vi "test-trajectory-generate-01.vi"() -> ()   [LabVIEW 2019]
uses:
  <vilib>/Rock Robotics/WPI/ThirdParty/JAS_Junk/TrajLib/Trajectory_Library.lvlib
  <vilib>/Rock Robotics/WPI/ThirdParty/JAS_Junk/TrajLib/TypeDef/TRANSLATION2D.ctl
  <vilib>/Rock Robotics/WPI/ThirdParty/JAS_Junk/TrajLib/TypeDef/ROTATION2D.ctl
  <vilib>/Rock Robotics/WPI/ThirdParty/JAS_Junk/TrajLib/TypeDef/POSE2D.ctl
  <vilib>/Rock Robotics/WPI/ThirdParty/JAS_Junk/TrajLib/TypeDef/TRAJ_STATE.ctl
panel:
  out "Accel\nExceeded (F)":bool
  out "Speed\nExceeded  (F)":bool
  out "TotalTImeSecs":dbl
  out "States":T1[](array[typedef]) {"POSE"."ROTATION"."SIN" format="%13.4f"; "POSE"."ROTATION"."COS" format="%13.4f"; "POSE"."ROTATION"."VALUE" format="%13.4f"; "POSE"."TRANSLATION"."Y" format="%14.3f"; "POSE"."TRANSLATION"."X" format="%14.3f"}
  out "XY Graph":cluster{dbl[], dbl[]}(graph)
  out "Numb\nWaypoints":i32
  out "All Interior \nwayPoints\nFound (True)":bool
  out "end rot = 0":dbl
  out "end y = 0":dbl
  out "end x = 0":dbl
  out "start rot = 0":dbl
  out "start y = 0":dbl
  out "start x = 0":dbl
  out "max dtheta < 0.0872":dbl
  out "max dy < 0.00127":dbl
  out "max dx  < 0.127":dbl
  out "Overall Error":errorcluster
  out "Elements":i32
  out "Elapsed Time":dbl
  # "THIS TEST SHOULD FAIL"
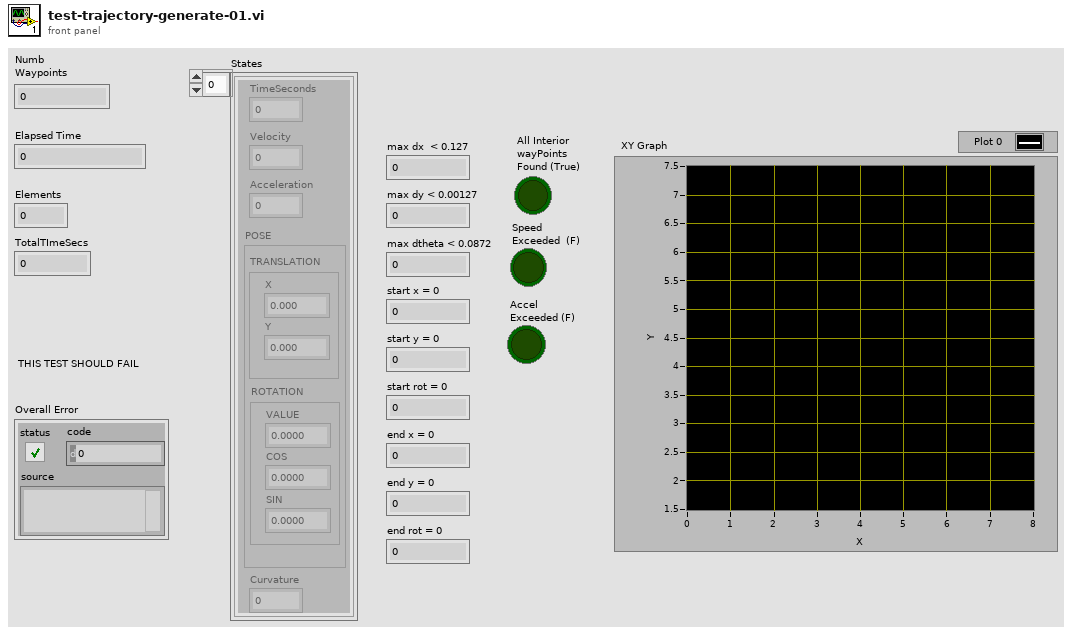
[diagram p1: front panel]
types:
  T1 = typedef "Trajectory_Library.lvlib/TRAJ_STATE.ctl" = cluster{"TimeSeconds":dbl, "Velocity":dbl, "Acceleration":dbl, "POSE":T2, "Curvature":dbl}
  T2 = typedef "Trajectory_Library.lvlib/POSE2D.ctl" = cluster{"TRANSLATION":T3, "ROTATION":T4}
  T3 = typedef "Trajectory_Library.lvlib/TRANSLATION2D.ctl" = cluster{"X":dbl, "Y":dbl}
  T4 = typedef "Trajectory_Library.lvlib/ROTATION2D.ctl" = cluster{"VALUE":dbl, "COS":dbl, "SIN":dbl}
  T5 = typedef "Trajectory_Library.lvlib/TRAJ_CONFIG.ctl" = cluster{"MaxVelocity":dbl, "Max Acceleration":dbl, "StartVelocity":dbl, "End Velocity":dbl, "Reversed":bool, "Constraints":variant[]}
  T6 = typedef "Trajectory_Library.lvlib/TRAJECTORY.ctl" = cluster{"TotalTImeSecs":dbl, "States":T1[]}
  T7 = typedef "Trajectory_Library.lvlib/TWIST2D.ctl" = cluster{"dX":dbl, "dY":dbl, "dTHETA":dbl}
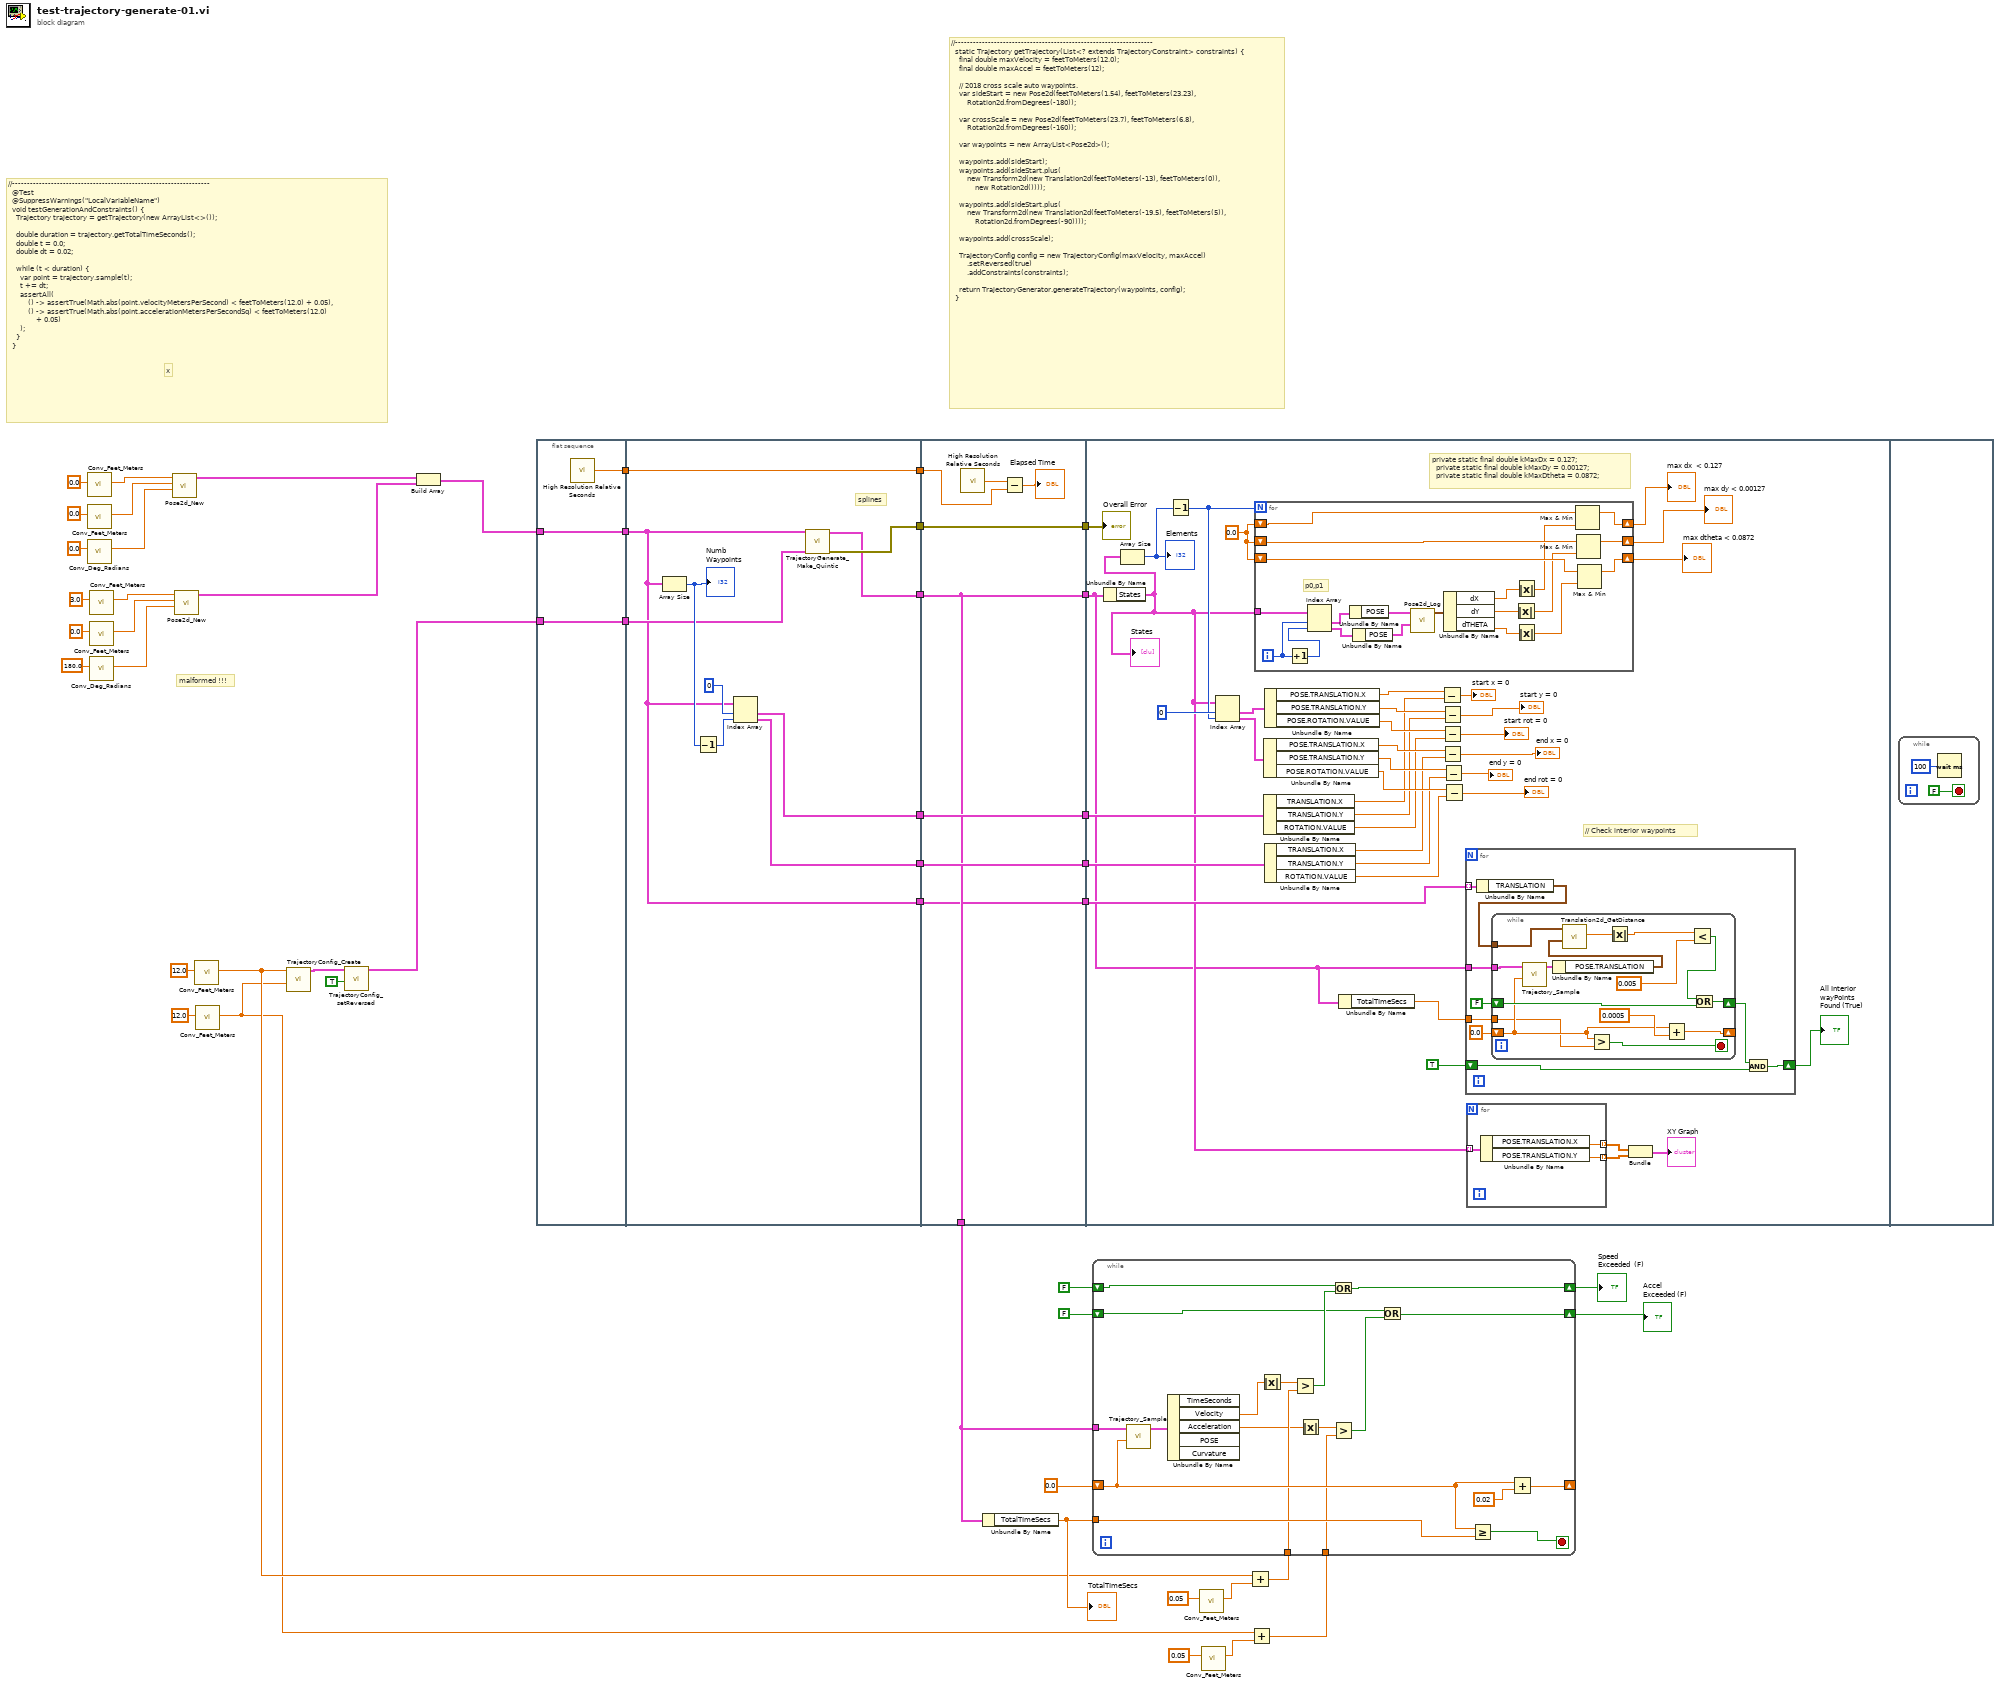
[diagram p0: block diagram]
diagram:
  # "malformed !!!"
  # "//------------------------------------------------------------------\n  @Test\n  @SuppressWarnings(\"LocalVariableName\")\n  void testGenerationAndConstraints() {\n    Trajectory trajectory = getTrajectory(new ArrayList<>());\n\n    double duration = trajectory.getTotalTimeSeconds();\n    double t = 0.0;\n    double dt = 0.02;\n\n    while (t < duration) {\n      var point = trajectory.sample(t);\n      t += dt;\n      assertAll(\n          () -> assertTrue(Math.abs(point.velocityMetersPerSecond) < feetToMeters(12.0) + 0.05),\n          () -> assertTrue(Math.abs(point.accelerationMetersPerSecondSq) < feetToMeters(12.0)\n              + 0.05)\n      );\n    }\n  }"
  # "//------------------------------------------------------------------\n  static Trajectory getTrajectory(List<? extends TrajectoryConstraint> constraints) {\n    final double maxVelocity = feetToMeters(12.0);\n    final double maxAccel = feetToMeters(12);\n\n    // 2018 cross scale auto waypoints.\n    var sideStart = new Pose2d(feetToMeters(1.54), feetToMeters(23.23),\n        Rotation2d.fromDegrees(-180));\n\n    var crossScale = new Pose2d(feetToMeters(23.7), feetToMeters(6.8),\n        Rotation2d.fromDegrees(-160));\n\n    var waypoints = new ArrayList<Pose2d>();\n\n    waypoints.add(sideStart);\n    waypoints.add(sideStart.plus(\n        new Transform2d(new Translation2d(feetToMeters(-13), feetToMeters(0)),\n            new Rotation2d())));\n\n    waypoints.add(sideStart.plus(\n        new Transform2d(new Translation2d(feetToMeters(-19.5), feetToMeters(5)),\n            Rotation2d.fromDegrees(-90))));\n\n    waypoints.add(crossScale);\n\n    TrajectoryConfig config = new TrajectoryConfig(maxVelocity, maxAccel)\n        .setReversed(true)\n        .addConstraints(constraints);\n\n    return TrajectoryGenerator.generateTrajectory(waypoints, config);\n  }"
  # "x"
  n1 = call <vilib>:"Conv_Feet_Meters.vi"("Feet"=0.0) -> ("Meters"=w39:dbl)  [unwired: 10 in]
  n2 = call <vilib>:"Conv_Feet_Meters.vi"("Feet"=0.0) -> ("Meters"=w38:dbl)  [unwired: 10 in]
  n3 = call <vilib>:"Conv_Deg_Radians.vi"("Degress"=0.0) -> ("Radians"=w37:dbl)  [unwired: 10 in]
  n4 = call <vilib>:"Conv_Feet_Meters.vi"("Feet"=3.0) -> ("Meters"=w33:dbl)  [unwired: 10 in]
  n5 = call <vilib>:"Conv_Feet_Meters.vi"("Feet"=0.0) -> ("Meters"=w32:dbl)  [unwired: 10 in]
  n6 = call <vilib>:"Conv_Deg_Radians.vi"("Degress"=180.0) -> ("Radians"=w31:dbl)  [unwired: 10 in]
  n7 = call <vilib>:"Pose2d_New.vi"("Heading"=w37, "Y"=w38, "X"=w39) -> ("out POSe"=w30:T2)  [unwired: 8 in]
  n8 = call <vilib>:"Pose2d_New.vi"("Heading"=w31, "Y"=w32, "X"=w33) -> ("out POSe"=w1:T2)  [unwired: 8 in]
  n9 = call <vilib>:"Conv_Feet_Meters.vi"("Feet"=12.0) -> ("Meters"=w14:dbl)  [unwired: 10 in]
  n10 = call <vilib>:"Conv_Feet_Meters.vi"("Feet"=12.0) -> ("Meters"=w4:dbl)  [unwired: 10 in]
  n11 = call <vilib>:"TrajectoryConfig_Create.vi"("MaxAcceleration"=w4, "MaxVelocity"=w14) -> ("TRAJECTORY_CONFIG"=w26:T5)  [unwired: 9 in]
  n12 = call <vilib>:"TrajectoryConfig_setReversed.vi"("Reversed"=TRUE, "inTRAJECTORY_CONFIG"=w26) -> ("outTRAJECTORY_CONFIG"=w22:T5)  [unwired: 9 in]
  n13 = Build Array(w30, w1) -> (w24:T2[])
  n14 = flat-sequence {
    tunnel: [w52] -> w49
    tunnel: [w51] -> w25
    tunnel: w24 -> [w51]
    tunnel: [w50] -> w23
    tunnel: w22 -> [w50]
    tunnel: [w62] -> w48
    tunnel: w49 -> [w62]
    tunnel: [w58] -> w46
    tunnel: [w57] -> w44
    tunnel: w25 -> [w53]
    tunnel: w23 -> [w54]
    tunnel: [w56] -> w21
    tunnel: [w55] -> w20
    tunnel: [w53] -> w2
    tunnel: w48 -> [w70]
    tunnel: [w65] -> w47
    tunnel: w46 -> [w67]
    tunnel: [w67] -> w45
    tunnel: w44 -> [w66]
    tunnel: [w66] -> w43
    tunnel: w21 -> [w65]
    tunnel: w20 -> [w64]
    tunnel: [w64] -> w19
    tunnel: [w64] -> w16
    tunnel: [w63] -> w3
    tunnel: w2 -> [w63]
    tunnel: w47 -> [w109]
    tunnel: w45 -> [w103]
    tunnel: w43 -> [w102]
    tunnel: w19 -> [w71]
    tunnel: w3 -> [w74]
    frame #0 {
      n15 = call <vilib>:"High Resolution Relative Seconds.vi"() -> ("relative seconds"=w52:dbl)
    }
    frame #1 {
      # "splines"
      n16 = Array Size(array=w53) -> (size(s)=w59:i32)
      "Numb\nWaypoints" <- w59
      n17 = Decrement(x=w59) -> (x-1=w60:i32)
      n18 = Index Array(array=w53, index #1=0 ("index"), index #2=w60) -> (element #1=w58:T2, element #2=w57:T2)
      n19 = call <vilib>:"TrajectoryGenerate_Make_Quintic.vi"("traj_config"=w54, "waypointPOSE"=w53) -> ("error out"=w56:errorcluster, "TRAJECTORY"=w55:T6)  [unwired: 8 in]
    }
    frame #2 {
      n20 = call <vilib>:"High Resolution Relative Seconds.vi"() -> ("relative seconds"=w68:dbl)
      n21 = Subtract(x=w68, y=w70) -> (x-y=→"Elapsed Time":dbl)
    }
    frame #3 {
      w107 = 0.0
      # "// Check interior waypoints"
      # "private static final double kMaxDx = 0.127;\n  private static final double kMaxDy = 0.00127;\n  private static final double kMaxDtheta = 0.0872;"
      n22 = Unbundle By Name(w71) -> ("States"=w72:T1[])
      "States" <- w72
      n23 = Array Size(array=w72) -> (size(s)=w108:i32)
      "Elements" <- w108
      n24 = Decrement(x=w108) -> (x-1=w100:i32)
      n25 = Index Array(array=w72, index #1=0 ("index"), index #2=w100) -> (element #1=w99:T1, element #2=w98:T1)
      n26 = for {
        N: w100 -> [_]
        tunnel: w72 -> [w154]
        shift-right: [w145] -> w106
        shift-left: w107 -> [w142]
        shift-right: [w143] -> w104
        shift-left: w107 -> [w140]
        shift-right: [w144] -> w105
        shift-left: w107 -> [w141]
        i -> [w156]
        # "p0,p1"
        n27 = Increment(x=w156) -> (x+1=w155:i32)
        n28 = Index Array(array=w154, index #1=w156, index #2=w155) -> (element #1=w153:T1, element #2=w152:T1)
        n29 = Unbundle By Name(w153) -> ("POSE"=w151:T2)
        n30 = Unbundle By Name(w152) -> ("POSE"=w150:T2)
        n31 = call <vilib>:"Pose2d_Log.vi"("end POSE"=w150, "in POSE"=w151) -> ("out TWIST"=w149:T7)  [unwired: 9 in]
        n32 = Unbundle By Name(w149) -> ("dX"=w146:dbl, "dY"=w147:dbl, "dTHETA"=w148:dbl)
        n33 = Absolute Value(x=w147) -> (abs(x)=w138:dbl)
        n34 = Absolute Value(x=w146) -> (abs(x)=w139:dbl)
        n35 = Absolute Value(x=w148) -> (abs(x)=w137:dbl)
        n36 = Max & Min(x=w142, y=w139) -> (max(x,y)=w145:dbl)  [unwired: 1 out]
        n37 = Max & Min(x=w141, y=w138) -> (max(x,y)=w144:dbl)  [unwired: 1 out]
        n38 = Max & Min(x=w140, y=w137) -> (max(x,y)=w143:dbl)  [unwired: 1 out]
      }
      "max dx  < 0.127" <- w106
      "max dy < 0.00127" <- w105
      "max dtheta < 0.0872" <- w104
      n39 = Unbundle By Name(w98) -> ("POSE.TRANSLATION.X"=w94:dbl, "POSE.TRANSLATION.Y"=w93:dbl, "POSE.ROTATION.VALUE"=w92:dbl)
      n40 = Unbundle By Name(w103) -> ("TRANSLATION.X"=w91:dbl, "TRANSLATION.Y"=w90:dbl, "ROTATION.VALUE"=w89:dbl)
      n41 = Unbundle By Name(w99) -> ("POSE.TRANSLATION.X"=w97:dbl, "POSE.TRANSLATION.Y"=w96:dbl, "POSE.ROTATION.VALUE"=w95:dbl)
      n42 = Unbundle By Name(w102) -> ("TRANSLATION.X"=w88:dbl, "TRANSLATION.Y"=w87:dbl, "ROTATION.VALUE"=w86:dbl)
      n43 = Unbundle By Name(w71) -> ("TotalTImeSecs"=w73:dbl)
      n44 = Subtract(x=w97, y=w91) -> (x-y=→"start x = 0":dbl)
      n45 = Subtract(x=w96, y=w90) -> (x-y=→"start y = 0":dbl)
      n46 = Subtract(x=w95, y=w89) -> (x-y=→"start rot = 0":dbl)
      n47 = Subtract(x=w94, y=w88) -> (x-y=→"end x = 0":dbl)
      n48 = Subtract(x=w93, y=w87) -> (x-y=→"end y = 0":dbl)
      n49 = Subtract(x=w92, y=w86) -> (x-y=→"end rot = 0":dbl)
      n50 = for {
        tunnel: w71 -> [w118]
        shift-right: [w117] -> w78
        shift-left: TRUE -> [w116]
        tunnel: w74 -> [w112] mode=indexing
        tunnel: w73 -> [w110]
        n51 = Unbundle By Name(w112) -> ("TRANSLATION"=w113:T3)
        n52 = while {
          tunnel: w118 -> [w127]
          shift-right: [w133] -> w114
          shift-left: FALSE -> [w132]
          tunnel: w113 -> [w131]
          shift-right: [w129] -> _
          shift-left: 0.0 -> [w121]
          tunnel: w110 -> [w120]
          stop <- w119 stop-if-true
          n53 = call <vilib>:"Trajectory_Sample.vi"("Time"=w121, "InputTRAJECTORY"=w127) -> ("OutputTRAJ_STATE"=w126:T1)  [unwired: 9 in]
          n54 = Unbundle By Name(w126) -> ("POSE.TRANSLATION"=w130:T3)
          n55 = call <vilib>:"Translation2d_GetDistance.vi"("other Translation"=w130, "In Translation"=w131) -> ("Distance"=w125:dbl)  [unwired: 9 in]
          n56 = Greater?(x=w121, y=w120) -> (0:w119:bool)
          n57 = Absolute Value(x=w125) -> (abs(x)=w124:dbl)
          n58 = Add(x=w121, y=0.0005) -> (x+y=w129:dbl)
          n59 = Less?(x=w124, y=0.005) -> (x < y?=w122:bool)
          n60 = Or(x=w122, y=w132) -> (x .or. y?=w133:bool)
        }
        n61 = And(x=w114, y=w116) -> (x .and. y?=w117:bool)
      }
      "All Interior \nwayPoints\nFound (True)" <- w78
      n62 = for {
        tunnel: [w136] -> w77 mode=indexing
        tunnel: [w135] -> w76 mode=indexing
        tunnel: w72 -> [w134] mode=indexing
        n63 = Unbundle By Name(w134) -> ("POSE.TRANSLATION.X"=w136:dbl, "POSE.TRANSLATION.Y"=w135:dbl)
      }
      n64 = Bundle(w77, w76) -> (→"XY Graph":cluster{dbl[], dbl[]})  [unwired: 1 in]
      "Overall Error" <- w109
    }
    frame #4 {
      n65 = while {
        stop <- FALSE stop-if-true
        n66 = Wait (ms)(milliseconds to wait=u32 100) -> ()  [unwired: 1 out]
      }
    }
  }
  n67 = Unbundle By Name(w16) -> ("TotalTImeSecs"=w17:dbl)
  "TotalTImeSecs" <- w17
  n68 = call <vilib>:"Conv_Feet_Meters.vi"("Feet"=0.05 ("y")) -> ("Meters"=w12:dbl)  [unwired: 10 in]
  n69 = call <vilib>:"Conv_Feet_Meters.vi"("Feet"=0.05 ("y")) -> ("Meters"=w9:dbl)  [unwired: 10 in]
  n70 = Add(x=w14, y=w12) -> (x+y=w11:dbl)
  n71 = Add(x=w4, y=w9) -> (x+y=w7:dbl)
  n72 = while {
    shift-right: [w176] -> _
    shift-left: 0.0 -> [w173]
    tunnel: w17 -> [w174]
    tunnel: w16 -> [w172]
    shift-right: [w168] -> w6
    shift-left: FALSE -> [w166]
    tunnel: w11 -> [w165]
    shift-right: [w161] -> w5
    shift-left: FALSE -> [w159]
    tunnel: w7 -> [w162]
    stop <- w175 stop-if-true
    n73 = call <vilib>:"Trajectory_Sample.vi"("Time"=w173, "InputTRAJECTORY"=w172) -> ("OutputTRAJ_STATE"=w171:T1)  [unwired: 9 in]
    n74 = Unbundle By Name(w171) -> ("Velocity"=w170:dbl, "Acceleration"=w163:dbl)  [unwired: 3 out]
    n75 = Absolute Value(x=w170) -> (abs(x)=w169:dbl)
    n76 = Greater?(x=w169, y=w165) -> (0:w167:bool)
    n77 = Absolute Value(x=w163) -> (abs(x)=w164:dbl)
    n78 = Or(x=w166, y=w167) -> (x .or. y?=w168:bool)
    n79 = Greater?(x=w164, y=w162) -> (0:w160:bool)
    n80 = Or(x=w159, y=w160) -> (x .or. y?=w161:bool)
    n81 = Greater Or Equal?(x=w173, y=w174) -> (x >= y?=w175:bool)
    n82 = Add(x=w173, y=0.02) -> (x+y=w176:dbl)
  }
  "Speed\nExceeded  (F)" <- w6
  "Accel\nExceeded (F)" <- w5
